vi "machine_parameters(SubVI).vi"(11 "error in (no error) 3":errorcluster) -> (0 "error out 3":errorcluster, 1 "Program name":string, 2 "Bolck of code being executed":string, 3 "Program status":string, 4 "Line of code":string, 5 "Machine availability":string, 6 "Emergency status":string, 7 "Controller mode":string)   [LabVIEW 2014]
uses:
  Program Files (x86)/National Instruments/LabVIEW 2014/vi.lib/addons/internet/NI_InternetTK_Core_VIs.lvlib
panel:
  out "error out 7":errorcluster
  out "error out 6":errorcluster
  out "error out 5":errorcluster
  out "error out 4":errorcluster
  out "error out 2":errorcluster
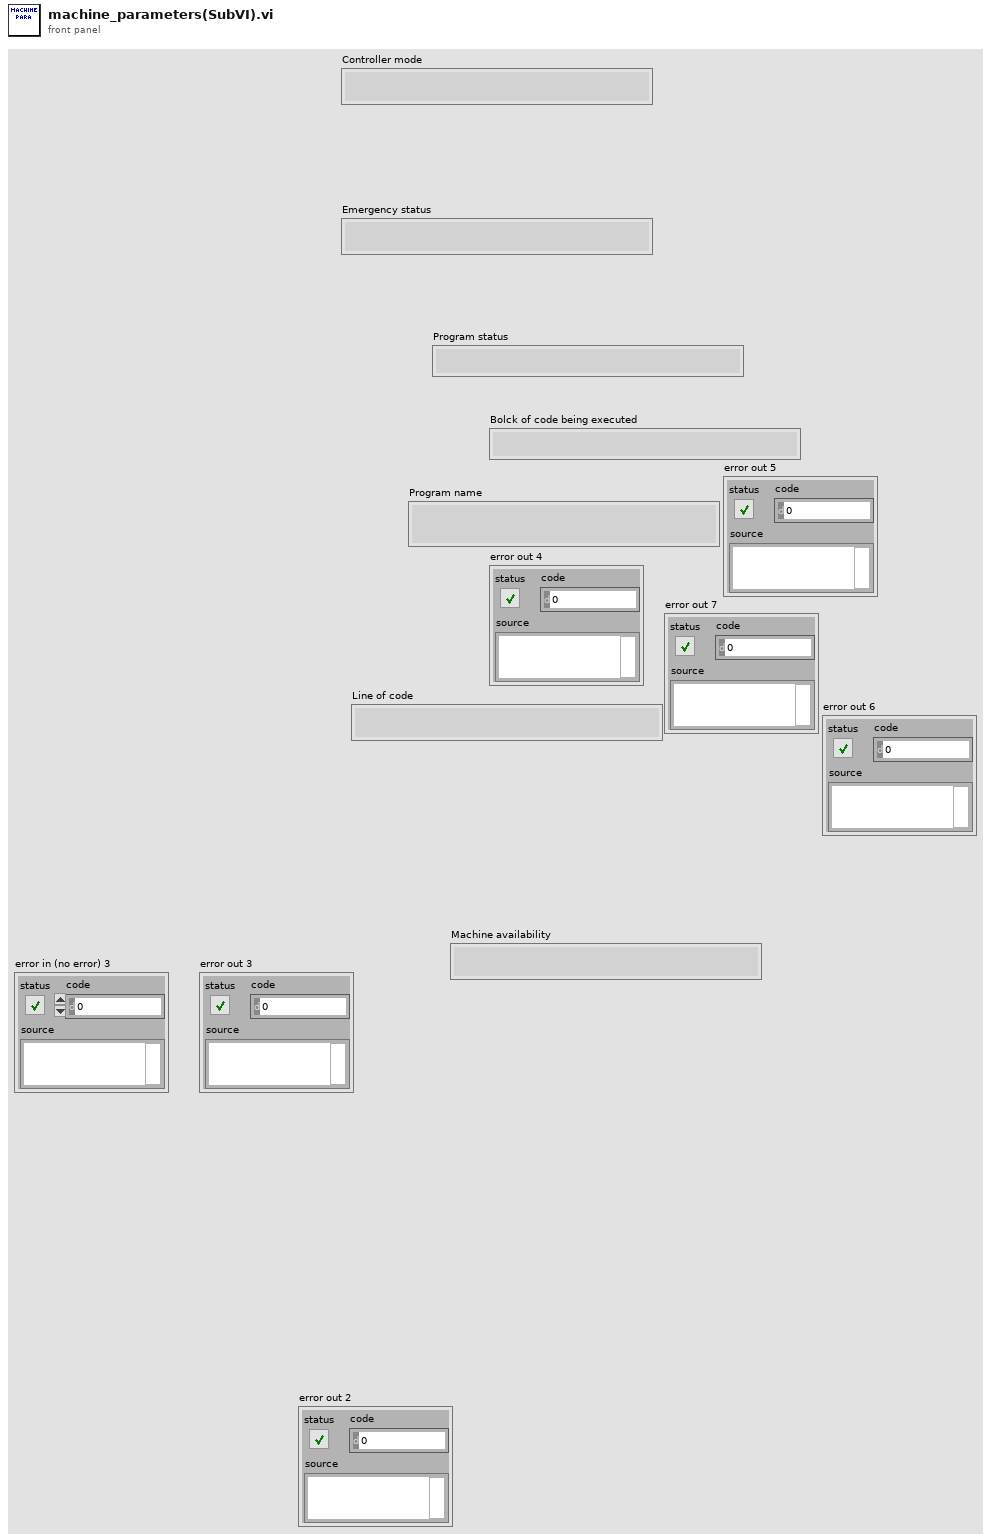
[diagram p1: front panel]
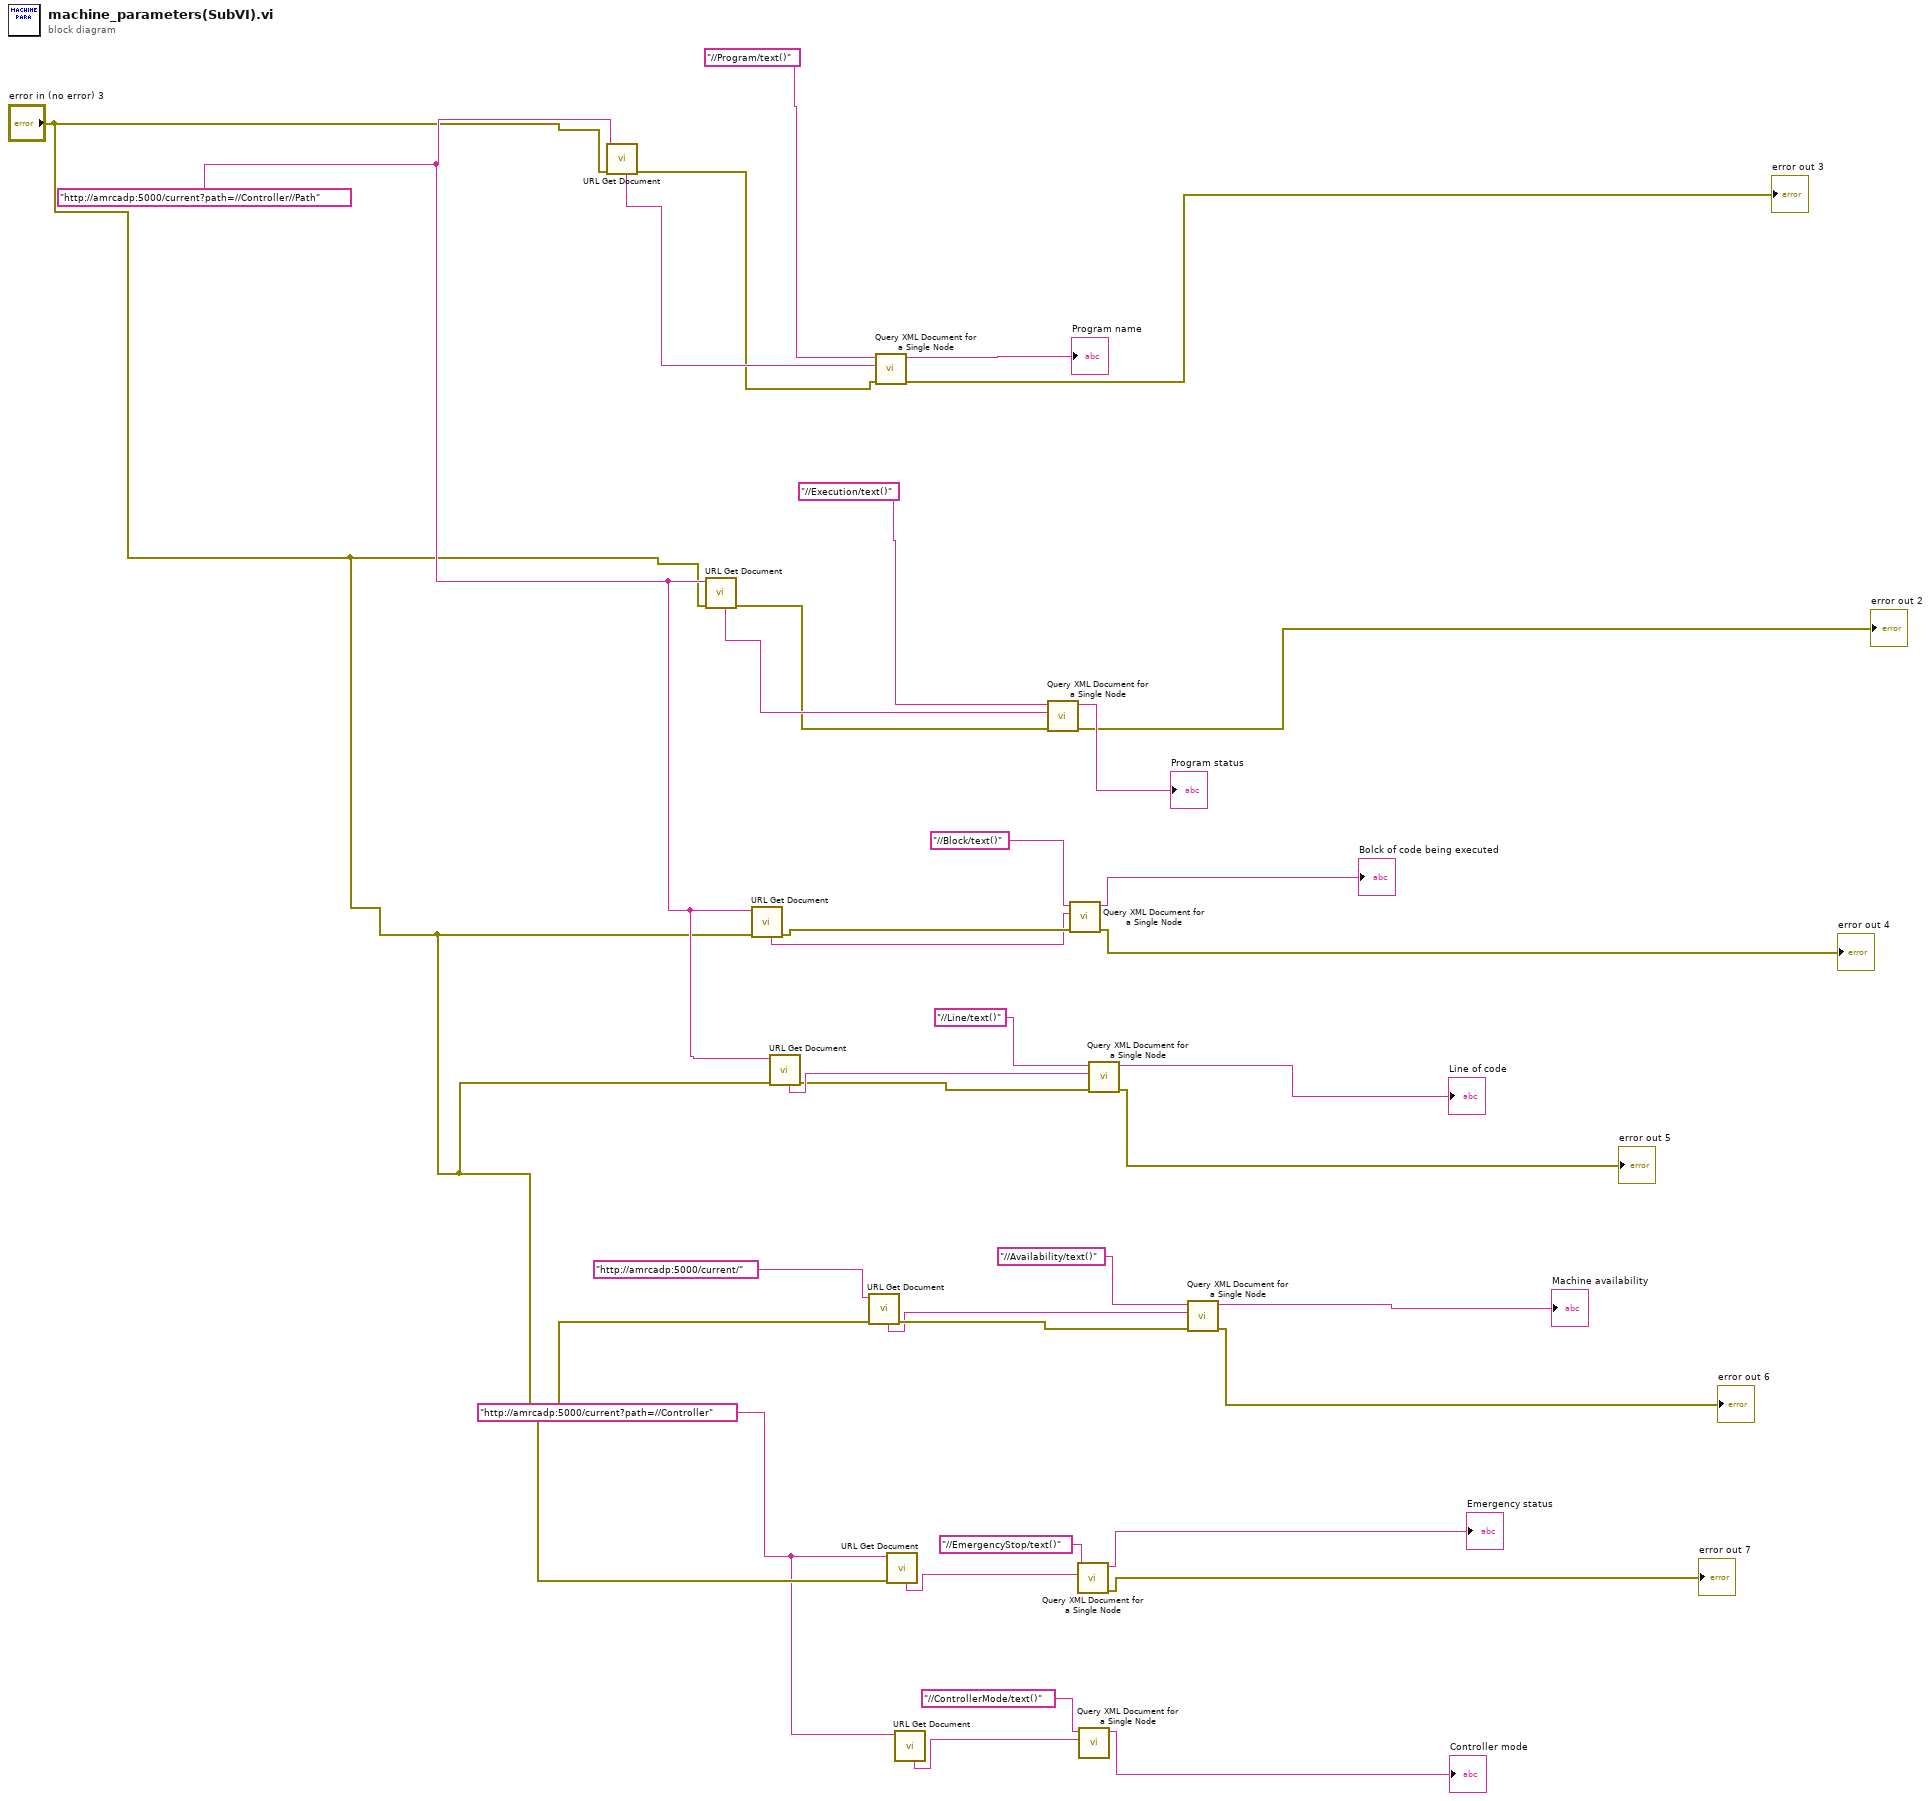
[diagram p0: block diagram]
diagram:
  w4 = "http://amrcadp:5000/current?path=//Controller" ("URL")
  w10 = "http://amrcadp:5000/current?path=//Controller//Path" ("URL")
  n1 = call "URL Get Document.vi"("error in (no error)"="error in (no error) 3", "URL"=w10) -> ("error out"=w28:errorcluster, "content"=w30:string)  [unwired: 5 in, 3 out]
  n2 = call "URL Get Document.vi"("error in (no error)"="error in (no error) 3", "URL"=w10) -> ("error out"=w27:errorcluster, "content"=w35:string)  [unwired: 5 in, 3 out]
  n3 = call "URL Get Document.vi"("error in (no error)"="error in (no error) 3", "URL"=w10) -> ("error out"=w26:errorcluster, "content"=w22:string)  [unwired: 5 in, 3 out]
  n4 = call "URL Get Document.vi"("error in (no error)"="error in (no error) 3", "URL"=w10) -> ("error out"=w17:errorcluster, "content"=w21:string)  [unwired: 5 in, 3 out]
  n5 = call "URL Get Document.vi"("error in (no error)"="error in (no error) 3", "URL"="http://amrcadp:5000/current/") -> ("error out"=w16:errorcluster, "content"=w12:string)  [unwired: 5 in, 3 out]
  n6 = call "Query XML Document for a Single Node.vi"("error in (no error)"=w28, "XML document"=w30, "XPath expression"="//Program/text()") -> ("error out"=→"error out 3":errorcluster, "Result XML"=→"Program name":string)  [unwired: 6 in, 1 out]
  n7 = call "URL Get Document.vi"("error in (no error)"="error in (no error) 3", "URL"=w4) -> ("content"=w9:string)  [unwired: 5 in, 4 out]
  n8 = call "URL Get Document.vi"("URL"=w4) -> ("content"=w3:string)  [unwired: 6 in, 4 out]
  n9 = call "Query XML Document for a Single Node.vi"("error in (no error)"=w27, "XML document"=w35, "XPath expression"="//Execution/text()") -> ("error out"=→"error out 2":errorcluster, "Result XML"=→"Program status":string)  [unwired: 6 in, 1 out]
  n10 = call "Query XML Document for a Single Node.vi"("error in (no error)"=w26, "XML document"=w22, "XPath expression"="//Block/text()") -> ("error out"=→"error out 4":errorcluster, "Result XML"=→"Bolck of code being executed":string)  [unwired: 6 in, 1 out]
  n11 = call "Query XML Document for a Single Node.vi"("XML document"=w9, "XPath expression"="//EmergencyStop/text()") -> ("error out"=→"error out 7":errorcluster, "Result XML"=→"Emergency status":string)  [unwired: 7 in, 1 out]
  n12 = call "Query XML Document for a Single Node.vi"("XML document"=w3, "XPath expression"="//ControllerMode/text()") -> ("Result XML"=→"Controller mode":string)  [unwired: 7 in, 2 out]
  n13 = call "Query XML Document for a Single Node.vi"("error in (no error)"=w17, "XML document"=w21, "XPath expression"="//Line/text()") -> ("error out"=→"error out 5":errorcluster, "Result XML"=→"Line of code":string)  [unwired: 6 in, 1 out]
  n14 = call "Query XML Document for a Single Node.vi"("error in (no error)"=w16, "XML document"=w12, "XPath expression"="//Availability/text()") -> ("error out"=→"error out 6":errorcluster, "Result XML"=→"Machine availability":string)  [unwired: 6 in, 1 out]
